vi "Picolog Get Temperatures.vi"(6 "Units":T1, 7 "Fill Missing Points":T2 items=["QNaN", "Previous"], 8 "Error In":errorcluster, 9 "Channels":i16[](array[numeric]), 10 "Buffer Length":i32, 11 "Instrument Handle In":i16) -> (0 "Error Out":errorcluster, 1 "Temperature":sgl[][](array[numeric]), 2 "Time [s]":dbl[][](array[numeric]), 3 "Instrument Handle Out":i16, 4 "Overflow":i16[](array[numeric]))   [LabVIEW 2017]
uses:
  Controls/Fill Missing.ctl
  Controls/Temperature Units.ctl
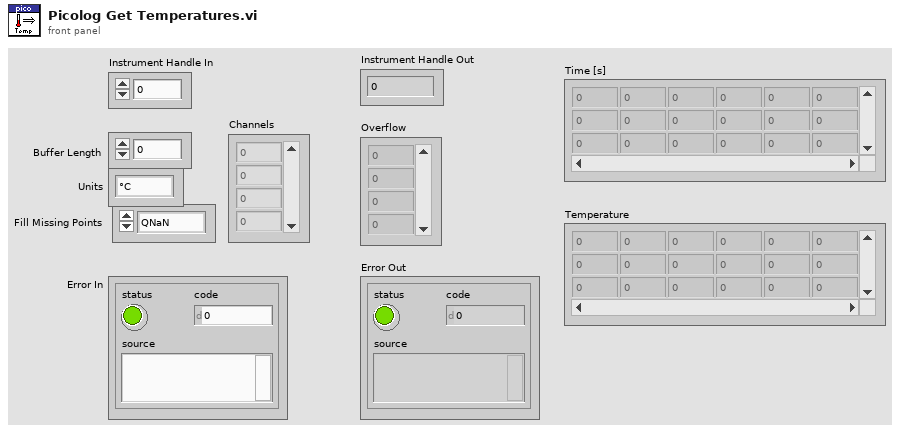
[diagram p1: front panel]
types:
  T1 = typedef "Temperature Units.ctl" = enum16{"°C", "°F", "K", "°R"}
  T2 = typedef "Fill Missing.ctl" = i16
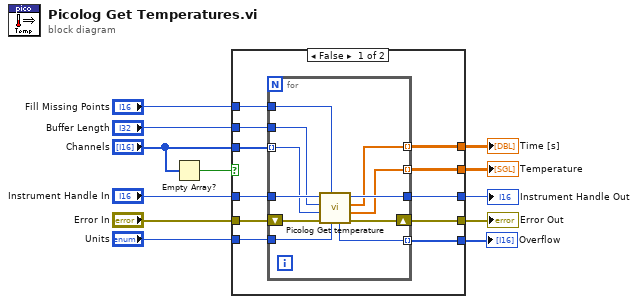
[diagram p0: block diagram]
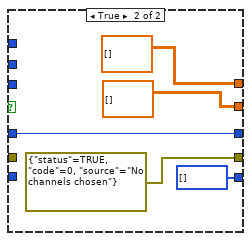
[diagram p2: hidden frame]
diagram:
  n1 = Empty Array?(array="Channels") -> (empty?=w2:bool)
  n2 = case shown="False" w2 {
    tunnel: [w23 sgl[][] [] ("Temperature")] -> w12
    tunnel: [w22 dbl[][] [] ("Time [s]")] -> w11
    tunnel: [w21 errorcluster {"status"=TRUE, "code"=0, "source"="No channels chosen"} ("Error In")] -> w10
    tunnel: "Buffer Length" -> [w20 _]
    tunnel: [w19 w36] -> w8
    tunnel: "Fill Missing Points" -> [w18 _]
    tunnel: "Units" -> [w17 _]
    tunnel: "Instrument Handle In" -> [w16 w36]
    tunnel: [w15 i16[] []] -> w4
    tunnel: "Channels" -> [w14 _]
    tunnel: "Error In" -> [w13 _]
    frame False {
      n3 = for {
        tunnel: w16 -> [w33]
        tunnel: w17 -> [w32]
        tunnel: w20 -> [w31]
        tunnel: w18 -> [w30]
        tunnel: [w29] -> w19
        tunnel: [w27] -> w22 mode=indexing
        tunnel: [w26] -> w23 mode=indexing
        shift-right: [w28] -> w21
        shift-left: w13 -> [w34]
        tunnel: w14 -> [w25] mode=indexing
        tunnel: [w24] -> w15 mode=indexing
        n4 = call "Picolog Get temperature.vi"("Units"=w32, "Fill Missing Points"=w30, "Error In"=w34, "Channel"=w25, "Buffer length"=w31, "Instrument Handle In"=w33) -> ("Error Out"=w28:errorcluster, "Temperature"=w26:sgl[], "Time [s]"=w27:dbl[], "Instrument Handle Out"=w29:i16, "Overflow"=w24:i16)  [unwired: 1 in]
      }
    }
    frame True {
    }
  }
  "Temperature" <- w12
  "Time [s]" <- w11
  "Error Out" <- w10
  "Instrument Handle Out" <- w8
  "Overflow" <- w4
